vi "nanocal-frontend-tcplink-client-LV19 -- V2.vi"() -> ()   [LabVIEW 2019]
doc: "Demonstrates how to open a connection to an TCP server, read the data being sent, and display the data on a chart. This VI is designed to stop if the TCP connection is terminated."
uses:
  nanocal server folder LV18/icicle.ctl
  nanocal server folder LV18/publisher action.ctl
panel:
  in  "Server Closed":string="The server VI closed the connection."
  in  "Tab Control":enum32{"Page 1", "Page 2"}(tab)
  in  "Stop":bool
  in  "address":string="146.201.231.45"
  in  "port":u16=6340
  in  "wait (ms)":u32=100
  out "nanocal data array OUT":T1[](array[typedef])
  # "nanocal tcplink --- client"
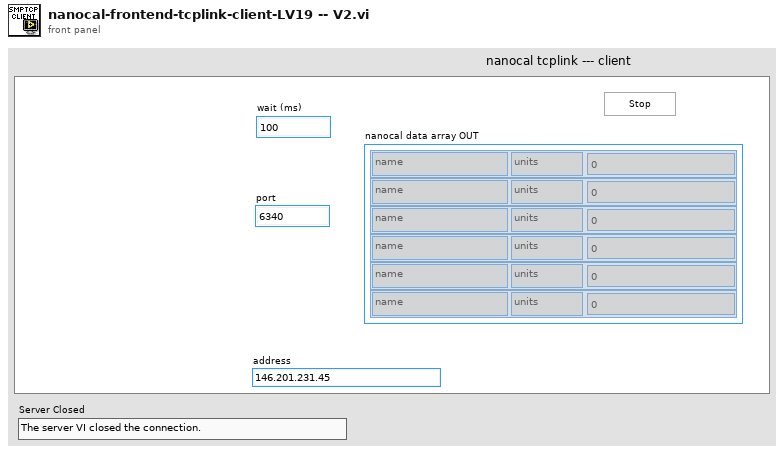
[diagram p1: front panel]
types:
  T1 = typedef "icicle.ctl" = cluster{"name":string, "units":string, "data":dbl}
  T2 = typedef "publisher action.ctl" = enum16{"set", "get", "init", "check"}
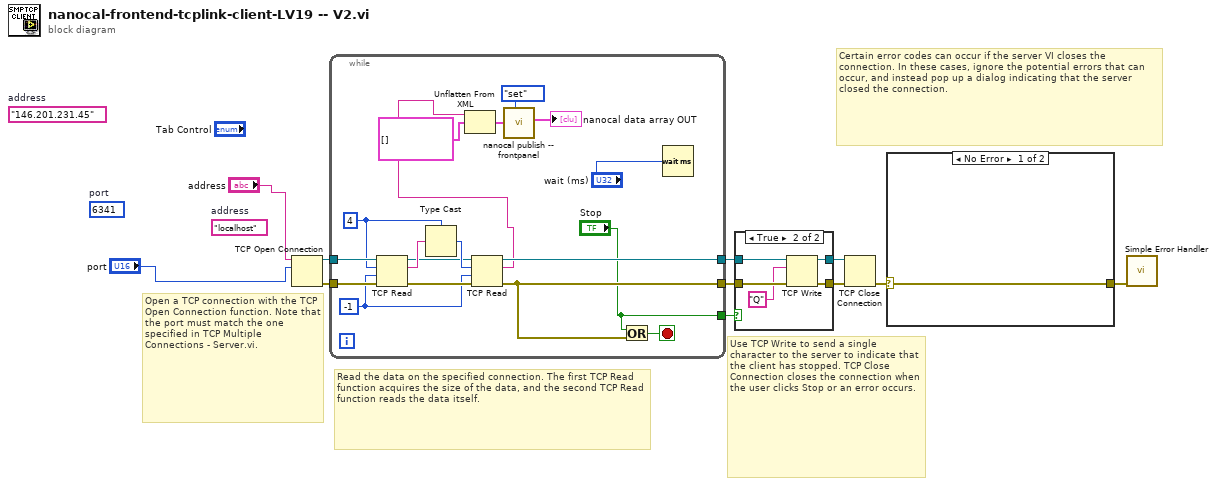
[diagram p0: block diagram]
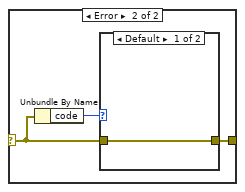
[diagram p2: hidden frame]
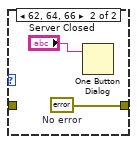
[diagram p3: hidden frame]
diagram:
  (unwired) u16 6341  # port
  (unwired) "localhost"  # address
  (unwired) "146.201.231.45"  # address
  # "Certain error codes can occur if the server VI closes the connection. In these cases, ignore the potential errors that can occur, and instead pop up a dialog indicating that the server closed the connection."
  # "Use TCP Write to send a single character to the server to indicate that the client has stopped. TCP Close Connection closes the connection when the user clicks Stop or an error occurs."
  # "Read the data on the specified connection. The first TCP Read function acquires the size of the data, and the second TCP Read function reads the data itself."
  # "Open a TCP connection with the TCP Open Connection function. Note that the port must match the one specified in TCP Multiple Connections - Server.vi."
  n1 = TCP Open Connection(address="address", remote port or service name="port") -> (connection ID=w11:refnum<k5>, error out=w10:errorcluster)  [unwired: 1 in, 2 out]
  n2 = while {
    tunnel: ["Stop"] -> w5
    tunnel: [w23] -> w9
    tunnel: [w21] -> w7
    tunnel: w10 -> [w28]
    tunnel: w11 -> [w29]
    stop <- w22 stop-if-true
    w19 = -1
    w20 = 4
    n3 = TCP Read(connection ID=w29, bytes to read=w20, error in (no error)=w28, 9:w19) -> (connection ID out=w24:refnum<k5>, data out=w27:string, error out=w26:errorcluster)  [unwired: 1 out]
    n4 = Type Cast(type=w20, x=w27) -> (*(type *) &x=w25:i32)
    n5 = TCP Read(connection ID=w24, bytes to read=w25, error in (no error)=w26, 9:w19) -> (connection ID out=w23:refnum<k5>, data out=w14:string, error out=w21:errorcluster)  [unwired: 1 out]
    n6 = Unflatten From XML(xml string=w14, type=T1[] []) -> (value=w16:T1[])  [unwired: 1 in, 1 out]
    n7 = call "nanocal publish -- frontpanel.vi"("publisher action"=publisher_action."set", "nanocal data array IN"=w16) -> ("nanocal data array OUT"=→"nanocal data array OUT":T1[])  [unwired: 9 in]
    n8 = Or(x="Stop", y=w21) -> (x .or. y?=w22:bool)
    n9 = Wait (ms)(milliseconds to wait="wait (ms)") -> ()  [unwired: 1 out]
  }
  n10 = case shown="True" w5 {
    tunnel: w9 -> [w31 w36]
    tunnel: [w31 w34] -> w8
    tunnel: w7 -> [w30 w35]
    tunnel: [w30 w33] -> w6
    frame False {
    }
    frame True {
      n11 = TCP Write(connection ID=w36, data in="Q", error in (no error)=w35) -> (connection ID out=w34:refnum<k5>, error out=w33:errorcluster)  [unwired: 2 out]
    }
  }
  n12 = TCP Close Connection(connection ID=w8, error in (no error)=w6) -> (error out=w4:errorcluster)  [unwired: 2 out]
  n13 = case shown="No Error" w4 {
    selector: w4 -> [w37 w39]
    tunnel: [w37 w38] -> w3
    frame No Error {
    }
    frame Error {
      n14 = Unbundle By Name(w39) -> ("code"=w40:i32)
      n15 = case shown="Default" w40 {
        tunnel: w39 -> [w41 _]
        tunnel: [w41 w43] -> w38
        frame Default {
        }
        frame 62, 64, 66 {
          w43 = errorcluster {"status"=FALSE, "code"=0, "source"=""}  # No error
          n16 = One Button Dialog(message="Server Closed") -> ()  [unwired: 1 in, 1 out]
        }
      }
    }
  }
  n17 = call <vilib>:"Simple Error Handler.vi"("error in (no error)"=w3) -> ()  [unwired: 1 in, 8 out]
